vi "XY Graph Bring Cursor To Center.vi"(8 "Error in":errorcluster caption="Error in (no error)", 9 "Active Cursor":u32, 11 "XY Graph Reference In":refnum<vi>) -> (0 "Error out":errorcluster, 3 "XY Graph Reference Out":refnum<vi>)   [LabVIEW 2024]
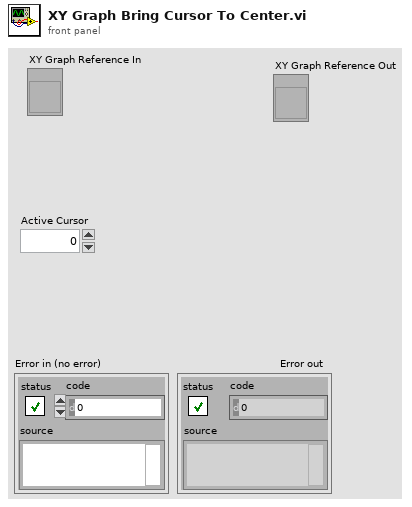
[diagram p1: front panel]
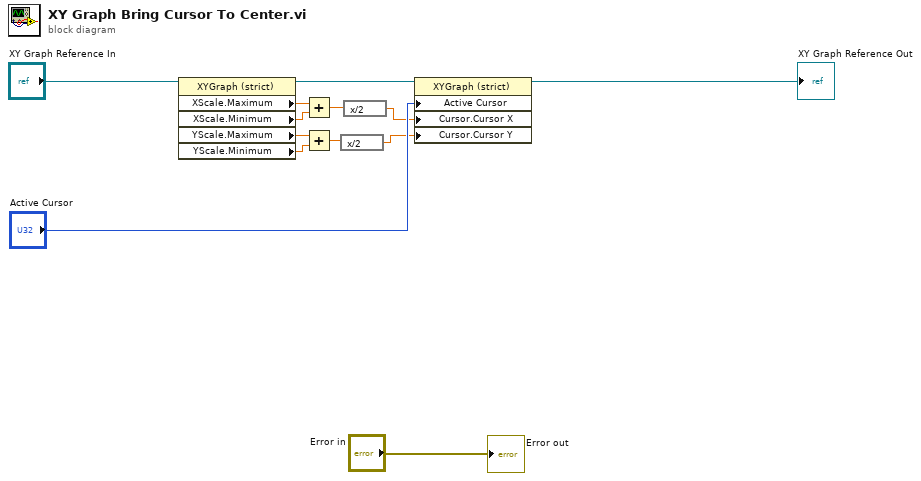
[diagram p0: block diagram]
diagram:
  n1 = property class="XYGraph (strict)"(reference="XY Graph Reference In") -> (reference out=w13:refnum<vi>, "XScale.Maximum"=w11:dbl, "XScale.Minimum"=w10:dbl, "YScale.Maximum"=w4:dbl, "YScale.Minimum"=w3:dbl)  [unwired: 1 in, 1 out]
  n2 = Add(x=w11, y=w10) -> (x+y=w5:dbl)
  n3 = Add(x=w4, y=w3) -> (x+y=w2:dbl)
  n4 = expression code="x/2"(w2) -> (w1:dbl)
  n5 = expression code="x/2"(w5) -> (w6:dbl)
  n6 = property class="XYGraph (strict)"(reference=w13, "Active Cursor"="Active Cursor", "Cursor.Cursor X"=w6, "Cursor.Cursor Y"=w1) -> (reference out=→"XY Graph Reference Out":refnum<vi>)  [unwired: 1 in, 1 out]
  "Error out" <- "Error in"
